vi "Image and data to image buffer FGV.vi"(6 "Current Calibration Parameters":T2, 8 "error in (no error)":errorcluster, 9 "AOL_Globals":T3 {"Angle Ys (degrees)" format="%#.6g"; "Angle Xs (degrees)" format="%#.6g"; "Plane Mode" items=["XY Plane", "XZ Plane", "YZ Plane", "arbitraryplane"]; "Frame Size" items=["100X100"=100, "128X128"=128, "200X200"=200, "256X256"=256, "512X512"=512, "1024x1024"=1024, "2048x2048"=2048]; "Back Apperture (mA)" format="%#.6g"; "Pockels (V)" format="%#.6g"; "PMT 2" format="%#.6g"; "PMT 1" format="%#.6g"; "Angle (degrees)" format="%#.6g"; "POI Dwell time (us)" format="%#.6g"}, 10 "Stage XYZ Position":cluster{"X":sgl, "Y":sgl, "Z":sgl}, 11 "Refnum in":T1) -> (0 "error out":errorcluster, 1 "LB data full":string[][](array[string]), 2 "LB data":string[][](array[string]), 3 "Refnum out":T1)   [LabVIEW 2020]
uses:
  Typedefs/Controls/AOL_Globals.ctl
  Typedefs/Imaging Protocols enum.ctl
  Typedefs/Frame Size.ctl
  Typedefs/AOL modes.ctl
  Typedefs/Plane Mode.ctl
  Typedefs/Functional Mode.ctl
  TypeDefs/Current Calibration Parameters.ctl
  <vilib>/vision/Image Controls.llb/IMAQ Image.ctl
  TypeDefs/data and image buffer fgv actions.ctl
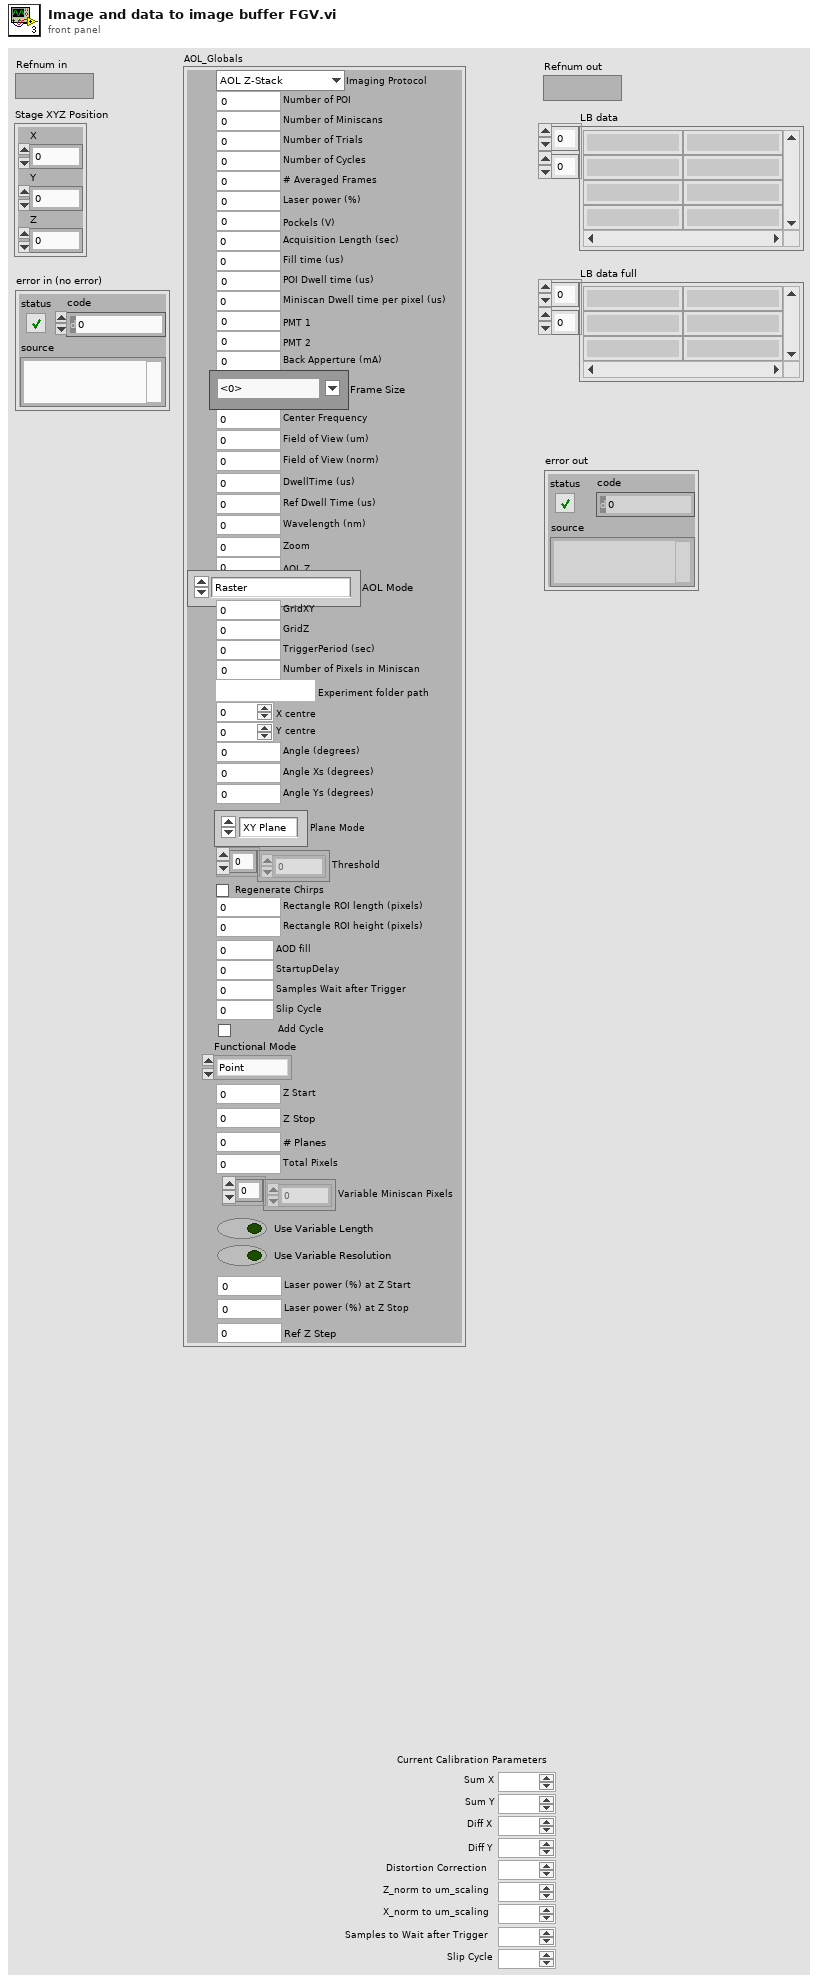
[diagram p1: front panel]
types:
  T1 = typedef "IMAQ Image.ctl" = refnum<image>
  T2 = typedef "Current Calibration Parameters.ctl" = cluster{"Sum X":dbl, "Sum Y":dbl, "Diff X":dbl, "Diff Y":dbl, "Distortion Correction":dbl, "Z_norm to um_scaling":dbl, "X_norm to um_scaling":dbl, "Samples to Wait after Trigger":dbl, "Slip Cycle":dbl}
  T3 = typedef "AOL_Globals.ctl" = cluster{"Imaging Protocol":T4, "Number of POI":u16, "Number of Miniscans":u16, "Number of Trials":u16, "Number of Cycles ":u64, "# Averaged Frames":u16, "Laser power (%)":u8, "Pockels (V)":dbl, "Acquisition Length (sec)":dbl, "Fill time (us)":dbl, "POI Dwell time (us)":dbl, "Miniscan Dwell time per pixel (us)":dbl, "PMT 1":dbl, "PMT 2":dbl, "Back Apperture (mA)":dbl, "Frame Size":T5, "Center Frequency":dbl, "Field of View (um)":dbl, "Field of View (norm)":dbl, "DwellTime (us)":dbl, "Ref Dwell Time (us)":dbl, "Wavelength (nm)":dbl, "Zoom":dbl, "AOL Z":dbl, "AOL Mode":T6, "GridXY":dbl, "GridZ":dbl, "TriggerPeriod (sec)":dbl, "Number of Pixels in Miniscan":u16, "Experiment folder path":path, "X centre":dbl, "Y centre":dbl, "Angle (degrees)":dbl, "Angle Xs (degrees)":dbl, "Angle Ys (degrees)":dbl, "Plane Mode":T7, "Threshold":u16[], "Regenerate Chirps":bool, "Rectangle ROI length (pixels)":u16, "Rectangle ROI height (pixels)":u16, "AOD fill":u16, "StartupDelay":i32, "Samples Wait after Trigger":u16, "Slip Cycle":u32, "Add Cycle":bool, "Functional Mode":T8, "Z Start":dbl, "Z Stop":dbl, "# Planes":i32, "Total Pixels":i32, "Variable Miniscan Pixels":u16[], "Use Variable Length":bool, "Use Variable Resolution":bool, "Laser power (%) at Z Start":u8, "Laser power (%) at Z Stop":u8, "Ref Z Step":i8}
  T4 = typedef "Imaging Protocols enum.ctl" = enum16{"AOL Z-Stack", "Motor Z Stack", "Parameter Sweep", "Functional Acquisition", "Single Plane Acquisition", "Volume Acquisition", "Live Imaging", "Live Plane Imaging", "Live Volume Imaging"}
  T5 = typedef "Frame Size.ctl" = u16
  T6 = typedef "AOL modes.ctl" = enum16{"Raster", "Structural", "Pointing", "Mini Scan", "Alignment"}
  T7 = typedef "Plane Mode.ctl" = u16
  T8 = typedef "Functional Mode.ctl" = enum16{"Point", "Line", "Patch", "Plane", "Volume"}
  T9 = typedef "data and image buffer fgv actions.ctl" = enum16{"Initialise", "Add Image to buffer", "Read Image buffer", "Edit specific data", "Delete selected image", "Clear all images"}
  T10 = typedef "Current Imaging Parameters.ctl" = cluster{"FOV":dbl, "Dwell Time":dbl, "Frame Size":dbl, "XPos":dbl, "YPos":dbl, "ZPos":dbl, "AOL-X":dbl, "AOL-Y":dbl, "AOL-Z":dbl, "X-Angle":dbl, "Y-Angle":dbl, "Z-Angle":dbl}
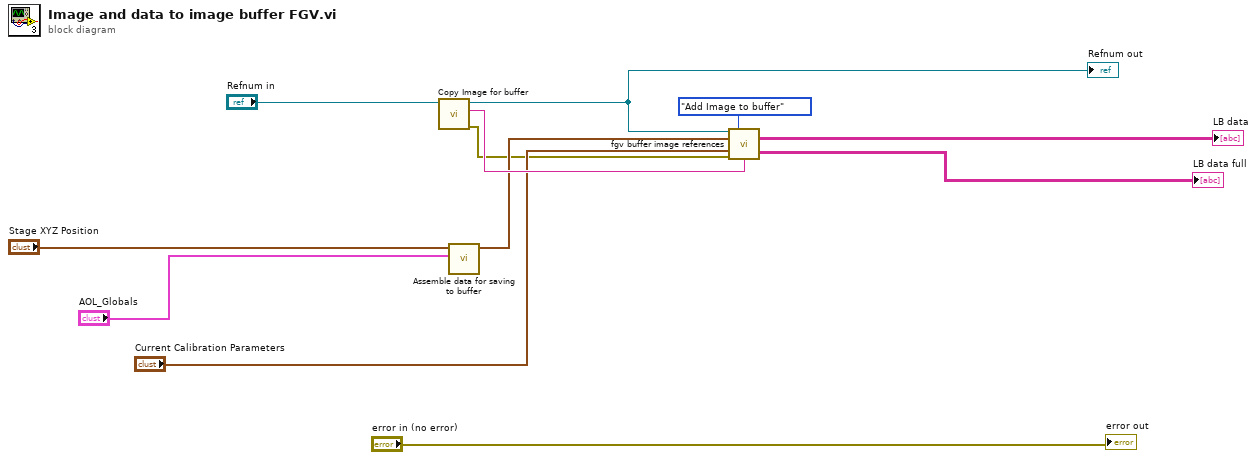
[diagram p0: block diagram]
diagram:
  n1 = call "Copy Image for buffer.vi"("Refnum in"="Refnum in") -> ("error out"=w3:errorcluster, "Image Name"=w9:string, "Refnum out"=w4:T1)  [unwired: 8 in]
  "Refnum out" <- w4
  n2 = call "Assemble data for saving to buffer.vi"("AOL_Globals"="AOL_Globals", "Stage XYZ Position"="Stage XYZ Position") -> ("Imaging Parameters"=w8:T10)  [unwired: 9 in]
  n3 = call "fgv buffer image references.vi"("Image Reference IN"=w4, "Actions"=data_and_image_buffer_fgv_actions."Add Image to buffer", "Imaging Parameters"=w8, "Calibration Parameters"="Current Calibration Parameters", "error in (no error)"=w3, "element"=w9) -> ("LB data"=→"LB data":string[][], "LB data full"=→"LB data full":string[][])  [unwired: 3 in, 5 out]
  "error out" <- "error in (no error)"
